vi "Initialize.vi"(4 "error in (no error)":errorcluster, 5 "Default setup (True)":bool=TRUE, 6 "ID Query (True)":bool=TRUE, 7 "VISA resource name":refnum<visa-resource-name>) -> (0 "error out":errorcluster, 1 "VISA resource name out":refnum<visa-resource-name>)   [LabVIEW 2017, in "GP22_TDC_Arduinoed.lvlib"]
doc: "Establishes communication with the instrument and optionally performs an instrument identification query and/or an instrument reset. It also places the instrument in a default state needed for other instrument driver operations. Therefore, call this VI before calling other instrument driver VIs for this instrument. Generally, you need to call the <b>Initialize</b> VI only once at the beginning of an application."
uses:
  GP22_TDC_Arduinoed.lvlib
panel:
  in  "Expected ID":string="GP22_DRIVER - 0.6"
  # "(c) 2014 <Enter Company Name Here>.  ALL RIGHTS RESERVED."
  # "EDIT: Change control description to remove example text for buses not supported."
  # "EDIT: Serial settings must match those on the physical instrument.  Review user's manual to determine the correct Flow Control protocol for the instrument.  \"None\" is the least robust option for this setting, and could lead to unreliable data transmission."
  # "EDIT: If your instrument does not support ID query or Reset, remove the ID Query or Reset control from the front panel and delete the case structure with the ID Query or Reset code from the block diagram."
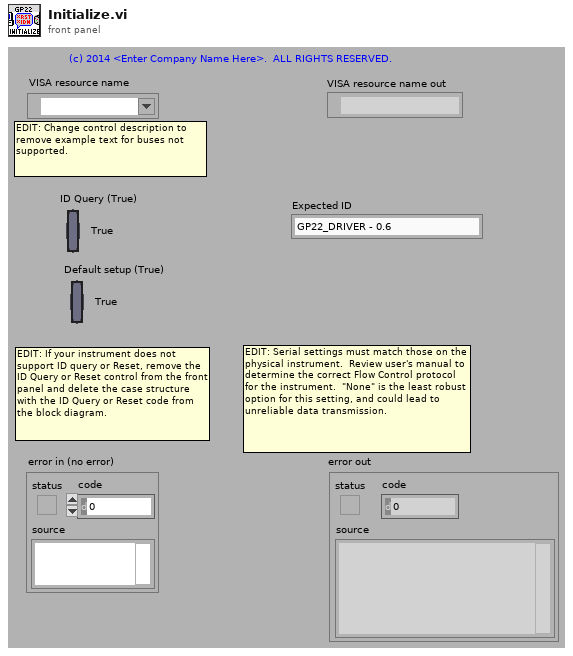
[diagram p1: front panel]
types:
  T1 = cluster{"Baud Rate":u32, "Parity":u16, "Data Bits":u16, "Stop Bits":u16, "Flow Control":u16}
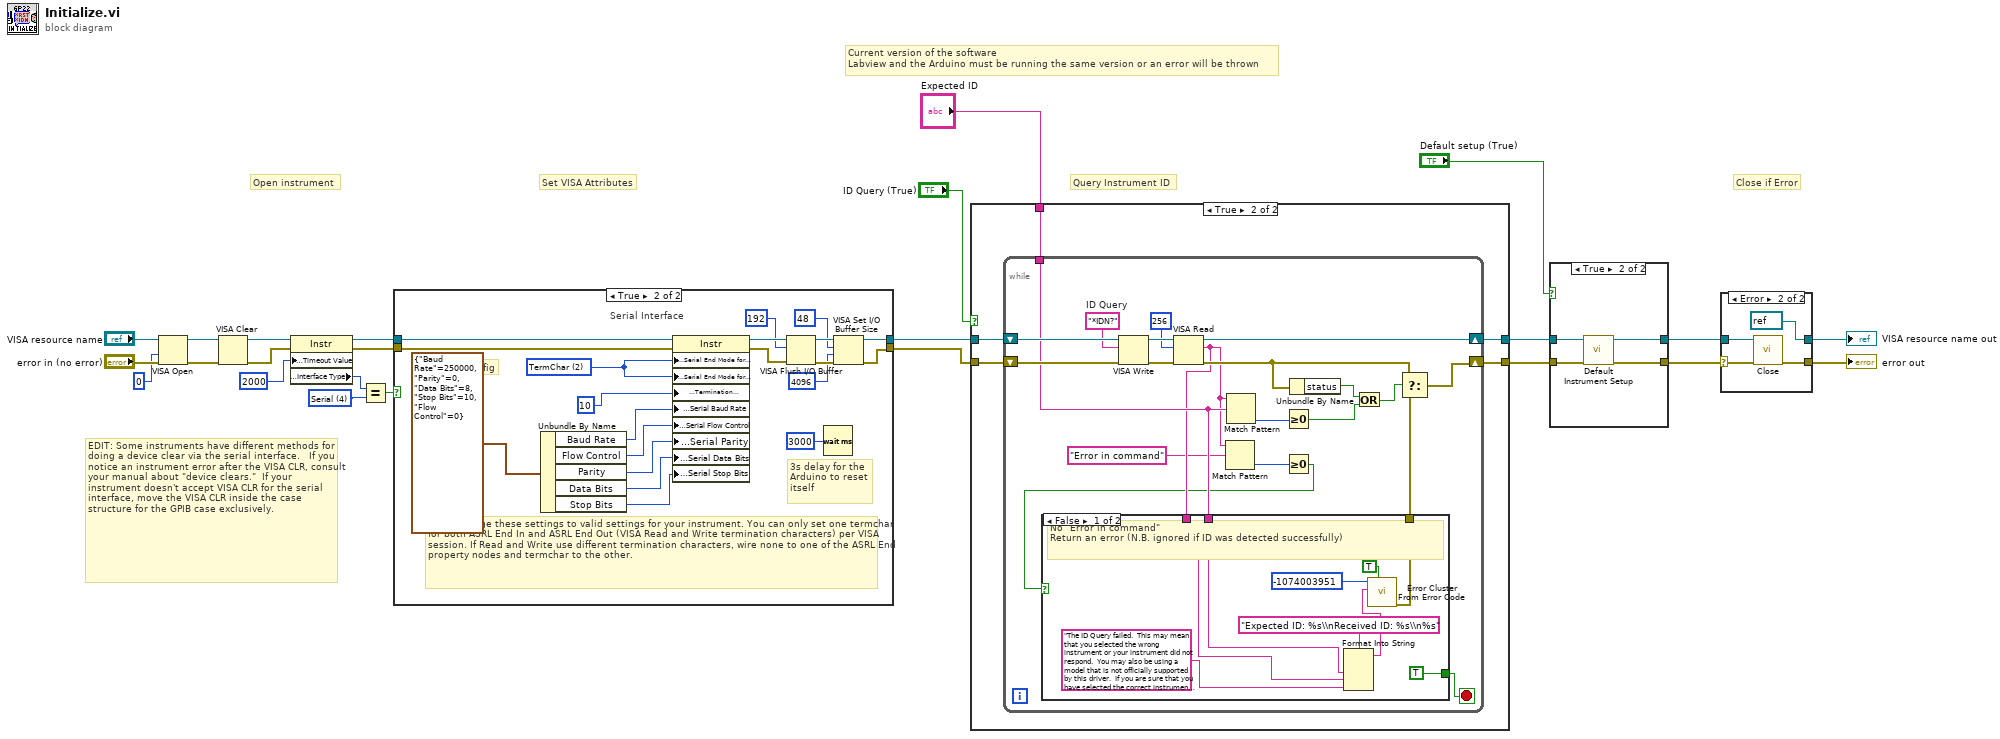
[diagram p0: block diagram]
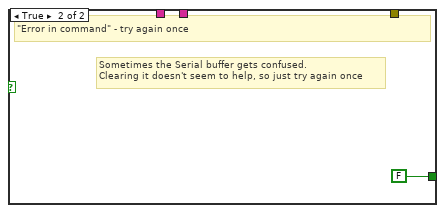
[diagram p6: hidden frame]
diagram:
  w12 = u16 4 items=["GPIB"=1, "VXI"=2, "GPIB-VXI"=3, "Serial"=4, "PXI"=5, "TCPIP"=6, "USB"=7] ("Interface Information:Interface Type")
  # "Current version of the software\nLabview and the Arduino must be running the same version or an error will be thrown"
  # "EDIT: Some instruments have different methods for doing a device clear via the serial interface.   If you notice an instrument error after the VISA CLR, consult your manual about \"device clears.\"  If your instrument doesn't accept VISA CLR for the serial interface, move the VISA CLR inside the case  structure for the GPIB case exclusively."
  # "Set VISA Attributes"
  # "Close if Error"
  # "Query Instrument ID"
  # "Open instrument"
  n1 = VISA Open(access mode=u32 0, error in (no error)="error in (no error)", VISA resource name="VISA resource name") -> (VISA resource name=w10:refnum<visa-resource-name>, error out=w9:errorcluster)  [unwired: 2 in]
  n2 = VISA Clear(VISA resource name=w10, error in (no error)=w9) -> (VISA resource name out=w8:refnum<visa-resource-name>, error out=w7:errorcluster)
  n3 = property class="Instr"(reference=w8, error in=w7, "General Settings:Timeout Value"=u32 2000) -> (reference out=w15:refnum<visa-resource-name>, error out=w14:errorcluster, "Interface Information:Interface Type"=w19:u16)
  n4 = Equal?(x=w19, y=w12) -> (x = y?=w13:bool)
  n5 = case shown="True" w13 {
    tunnel: [w25 w43] -> w17
    tunnel: [w26 w40] -> w16
    tunnel: w15 -> [w25 w45]
    tunnel: w14 -> [w26 w46]
    frame False {
      # "EDIT: Remove interfaces not supported by your instrument."
      # "GPIB, TCP/IP, and USB Interface"
    }
    frame True {
      w35 = u16 2 items=["None", "LastBit", "TermChar"] ("Serial Settings:Serial End Mode for Reads")
      # "3s delay for the\nArduino to reset\nitself"
      # "Serial config"
      # "EDIT: Change these settings to valid settings for your instrument. You can only set one termchar for both ASRL End In and ASRL End Out (VISA Read and Write termination characters) per VISA session. If Read and Write use different termination characters, wire none to one of the ASRL End property nodes and termchar to the other."
      # "Serial Interface"
      n6 = Unbundle By Name(T1 {"Baud Rate"=250000, "Parity"=0, "Data Bits"=8, "Stop Bits"=10, "Flow Control"=0} ("Serial Configuration")) -> ("Baud Rate"=w34:u32, "Flow Control"=w30:u16, "Parity"=w32:u16, "Data Bits"=w33:u16, "Stop Bits"=w29:u16)
      n7 = property class="Instr"(reference=w45, error in=w46, "Serial Settings:Serial End Mode for Reads"=w35, "Serial Settings:Serial End Mode for Writes"=w35, "Message Based Settings:Termination Character"=u8 10, "Serial Settings:Serial Baud Rate"=w34, "Serial Settings:Serial Flow Control"=w30, "Serial Settings:Serial Parity"=w32, "Serial Settings:Serial Data Bits"=w33, "Serial Settings:Serial Stop Bits"=w29) -> (reference out=w39:refnum<visa-resource-name>, error out=w42:errorcluster)
      n8 = VISA Flush I/O Buffer(VISA resource name=w39, mask (16)=u16 192, error in (no error)=w42) -> (VISA resource name out=w44:refnum<visa-resource-name>, error out=w41:errorcluster)
      n9 = Wait (ms)(milliseconds to wait=u32 3000) -> ()  [unwired: 1 out]
      n10 = VISA Set I/O Buffer Size(VISA resource name=w44, mask (16)=u16 48, size (4096)=u32 4096 ("size (0)"), error in (no error)=w41) -> (VISA resource name out=w43:refnum<visa-resource-name>, error out=w40:errorcluster)
    }
  }
  n11 = case shown="True" "ID Query (True)" {
    tunnel: [w47 w53] -> w23
    tunnel: [w48 w50] -> w24
    tunnel: w17 -> [w48 w51]
    tunnel: w16 -> [w47 w52]
    tunnel: "Expected ID" -> [_ w49]
    frame False {
    }
    frame True {
      n12 = while {
        tunnel: w49 -> [w69]
        shift-right: [w73] -> w53
        shift-left: w52 -> [w72]
        shift-right: [w70] -> w50
        shift-left: w51 -> [w71]
        stop <- w54 stop-if-true
        w65 = "*IDN?"  # ID Query
        n13 = VISA Write(VISA resource name=w71, write buffer=w65, error in (no error)=w72) -> (VISA resource name out=w68:refnum<visa-resource-name>, error out=w67:errorcluster)  [unwired: 1 out]
        n14 = VISA Read(VISA resource name=w68, byte count=u32 256, error in (no error)=w67) -> (VISA resource name out=w70:refnum<visa-resource-name>, read buffer=w58:string, error out=w63:errorcluster)  [unwired: 1 out]
        n15 = Match Pattern(string=w58, regular expression="Error in command") -> (offset past match=w56:i32)  [unwired: 1 in, 3 out]
        n16 = Match Pattern(string=w58, regular expression=w69) -> (offset past match=w64:i32)  [unwired: 1 in, 3 out]
        n17 = Greater Or Equal To 0?(x=w64) -> (x >= 0?=w61:bool)
        n18 = Greater Or Equal To 0?(x=w56) -> (x >= 0?=w55:bool)
        n19 = case shown="False" w55 {
          tunnel: w69 -> [w82 _]
          tunnel: [w76 _] -> w59
          tunnel: w58 -> [w75 _]
          tunnel: [TRUE FALSE] -> w54
          frame False {
            # "No \"Error in command\"\nReturn an error (N.B. ignored if ID was detected successfully)"
            n20 = Format Into String(format string="Expected ID: %s\\nReceived ID: %s\\n%s", w82, w75, "The ID Query failed.  This may mean that you selected the wrong instrument or your instrument did not respond.  You may also be using a model that is not officially supported by this driver.  If you are sure that you have selected the correct instrument and it is responding, try disabling the ID Query." ("Source (VI Name)")) -> (resulting string=w79:string)  [unwired: 2 in, 1 out]
            n21 = call <vilib>:"Error Cluster From Error Code.vi"("show call chain? (False)"=TRUE, "error message (\"\")"=w79, "error code (0)"=-1074003951 ("Code")) -> ("error out"=w76:errorcluster)  [unwired: 6 in]
          }
          frame True {
            # "Sometimes the Serial buffer gets confused. \nClearing it doesn't seem to help, so just try again once"
            # "\"Error in command\" - try again once"
          }
        }
        n22 = Unbundle By Name(w63) -> ("status"=w62:bool)
        n23 = Or(x=w62, y=w61) -> (x .or. y?=w60:bool)
        n24 = Select(t=w63, s=w60, f=w59) -> (s? t:f=w73:errorcluster)
      }
    }
  }
  n25 = case shown="True" "Default setup (True)" {
    tunnel: w24 -> [w85 w89]
    tunnel: w23 -> [w84 w88]
    tunnel: [w85 w87] -> w4
    tunnel: [w84 w86] -> w3
    frame False {
    }
    frame True {
      n26 = call "Default Instrument Setup.vi"("error in (no error)"=w88, "VISA resource name"=w89) -> ("error out"=w86:errorcluster, "VISA resource name out"=w87:refnum<visa-resource-name>)  [unwired: 8 in]
    }
  }
  n27 = case shown="Error" w3 {
    selector: w3 -> [w90 w93]
    tunnel: w4 -> [w91 w94]
    tunnel: [w91 refnum<visa-resource-name> refnum ("VISA resource name out")] -> w6
    tunnel: [w90 w95] -> w5
    frame No Error {
    }
    frame Error {
      n28 = call "Close.vi"("error in (no error)"=w93, "VISA resource name"=w94) -> ("error out"=w95:errorcluster)  [unwired: 9 in]
    }
  }
  "VISA resource name out" <- w6
  "error out" <- w5
